vi "Move ListSelection.vi"(4 "Bias":i32, 6 "Size":i32, 7 "Herizon":i32, 8 "error in (no error)":errorcluster, 9 "List_Rec":T1, 10 "Mou_Pos":T1, 11 "ListSelection in":refnum<class "ListSelection.lvclass">) -> (0 "error out":errorcluster, 3 "ListSelection out":refnum<class "ListSelection.lvclass">)   [LabVIEW 2015, in "Admin_Actor.lvlib" / "ListSelection.lvclass"]
uses:
  ListSelection.lvclass
  <vilib>/Utility/miscctls.llb/LVPositionTypeDef.ctl
  ListSelection.lvclass/ListSelection.ctl
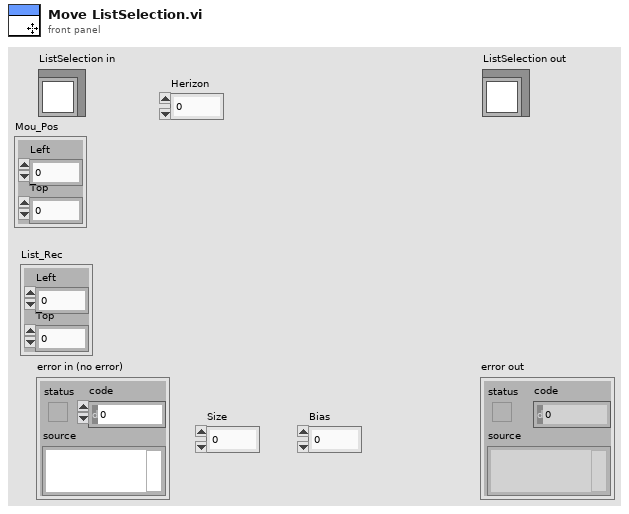
[diagram p1: front panel]
types:
  T1 = typedef "LVPositionTypeDef.ctl" = cluster{"Left":i32, "Top":i32}
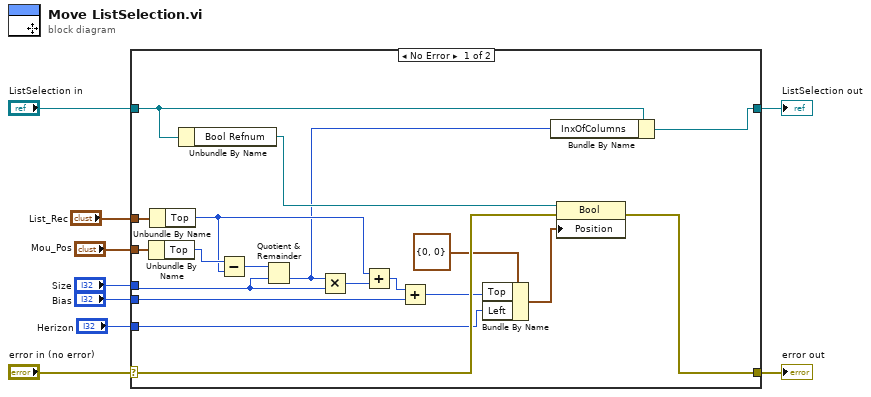
[diagram p0: block diagram]
diagram:
  n1 = case shown="No Error" "error in (no error)" {
    selector: "error in (no error)" -> [w27 w30]
    tunnel: [w13 w30] -> w8
    tunnel: [w10 w29] -> w6
    tunnel: "ListSelection in" -> [w12 w29]
    tunnel: "List_Rec" -> [w25 _]
    tunnel: "Mou_Pos" -> [w24 _]
    tunnel: "Size" -> [w19 _]
    tunnel: "Bias" -> [w18 _]
    tunnel: "Herizon" -> [w15 _]
    frame No Error {
      n2 = Unbundle By Name(w24) -> ("Top"=w23:i32)
      n3 = Unbundle By Name(w25) -> ("Top"=w20:i32)
      n4 = Unbundle By Name(w12) -> ("Bool Refnum"=w28:refnum<vi>)
      n5 = Subtract(x=w23, y=w20) -> (x-y=w26:i32)
      n6 = Quotient & Remainder(x=w26, y=w19) -> (floor(x/y)=w11:i32)  [unwired: 1 out]
      n7 = Multiply(x=w11, y=w19) -> (x*y=w21:i32)
      n8 = Add(x=w20, y=w21) -> (x+y=w22:i32)
      n9 = Add(x=w22, y=w18) -> (x+y=w16:i32)
      n10 = Bundle By Name(cluster=T1 {"Left"=0, "Top"=0} ("Position"), "Top"=w16, "Left"=w15) -> (w14:T1)
      n11 = Bundle By Name(cluster=w12, "InxOfColumns"=w11) -> (w10:refnum<class "ListSelection.lvclass">)
      n12 = property class="Bool"(reference=w28, error in=w27, "Position"=w14) -> (error out=w13:errorcluster)  [unwired: 1 out]
    }
    frame Error {
    }
  }
  "error out" <- w8
  "ListSelection out" <- w6
